vi "MIC.vi"() -> ()   [LabVIEW 2022 SP3]
uses:
  <vilib>/Analysis/3filter.llb/Filter Passband Type.ctl
  <vilib>/DAQmx/read.llb/DAQmx Read (Analog 1D Wfm NChan NSamp).vi
  <vilib>/DAQmx/write.llb/DAQmx Write (Analog 1D DBL NChan 1Samp).vi
  <vilib>/DAQmx/create/channels.llb/DAQmx Create Channel (AI-Voltage-Basic).vi
  <vilib>/DAQmx/configure/timing.llb/DAQmx Timing (Sample Clock).vi
  <vilib>/DAQmx/create/channels.llb/DAQmx Create Channel (AO-Voltage-Basic).vi
  <vilib>/DAQmx/miscellaneous.llb/DAQmx Fill In Error Info.vi
  <vilib>/Analysis/3filter.llb/Butterworth Filter (DBL).vi
  <vilib>/Analysis/NI_AALBase.lvlib
panel:
  out "Inverted Signal":dbl[](graph)
  out "Y":dbl[](array[numeric])
  in  "stop":bool
  out "Filtered":dbl[](graph)
  out "Filtered X":dbl[](array[numeric])
  out "INput":dbl[](graph)
  out "data":waveform(dbl)
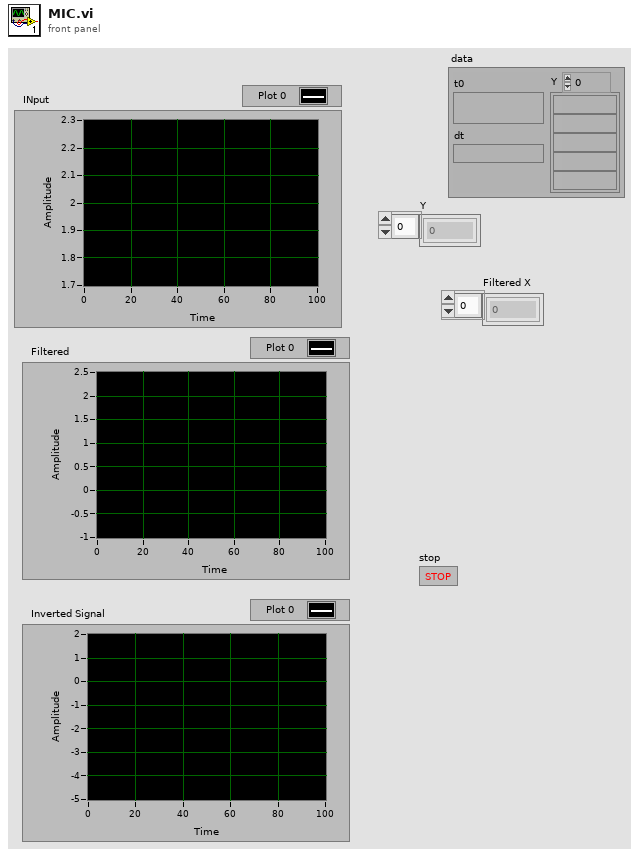
[diagram p1: front panel]
types:
  T1 = typedef "NI_AALBase.lvlib/Filter Passband Type.ctl" = enum32{"Lowpass", "Highpass", "Bandpass", "Bandstop"}
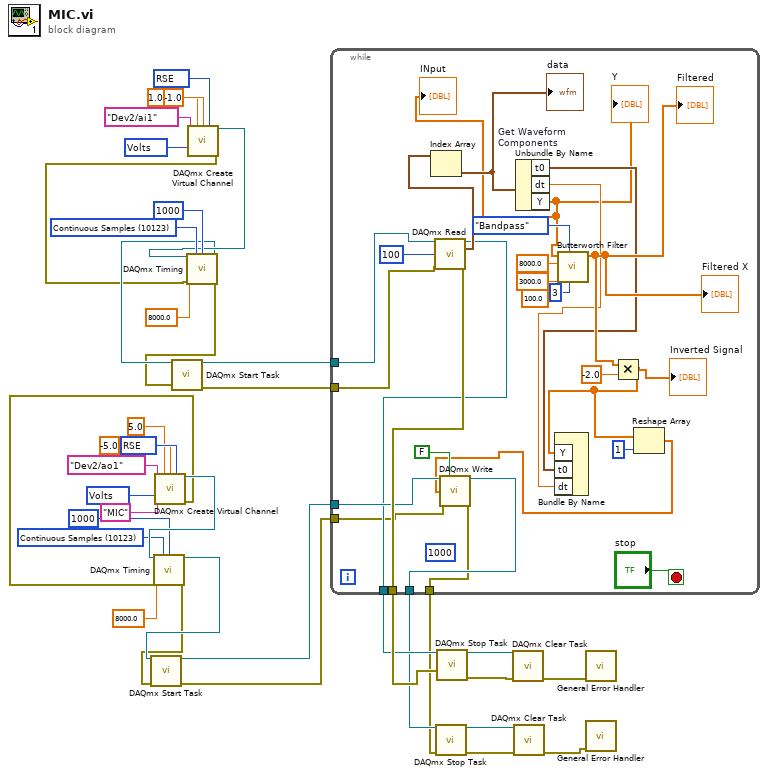
[diagram p0: block diagram]
diagram:
  w14 = 10123 items=["Finite Samples"=10178, "Continuous Samples"=10123, "Hardware Timed Single Point"=12522] ("sample mode")
  w18 = 10083 items=["Default"=-1, "RSE"=10083, "Differential"=10106, "Pseudodifferential"=12529] ("output terminal configuration")
  w20 = 10348 items=["Volts"=10348, "From Custom Scale"=10065] ("units")
  w32 = 10083 items=["Default"=-1, "RSE"=10083, "NRSE"=10078, "Differential"=10106, "Pseudodifferential"=12529] ("input terminal configuration")
  w33 = 10348 items=["Volts"=10348, "From Custom Scale"=10065] ("units")
  w35 = 10123 items=["Finite Samples"=10178, "Continuous Samples"=10123, "Hardware Timed Single Point"=12522] ("sample mode")
  n1 = call-poly <vilib>:"DAQmx Create Virtual Channel.vi"("maximum value"=5.0, "minimum value"=-5.0, "output terminal configuration"=w18, "physical channels"=tag "Dev2/ao1", "name to assign"="MIC", "units"=w20) -> ("task out"=w15:refnum<k21>, "error out"=w11:errorcluster)  [unwired: 8 in]
  n2 = call-poly <vilib>:"DAQmx Timing.vi"("task/channels in"=w15, "sample mode"=w14, "samples per channel"=1000, "rate"=8000.0, "error in"=w11) -> ("task out"=w10:refnum<k21>, "error out"=w5:errorcluster)  [unwired: 9 in]
  n3 = call <vilib>:"DAQmx Start Task.vi"("task/channels in"=w10, "error in"=w5) -> ("task out"=w9:refnum<k21>, "error out"=w4:errorcluster)  [unwired: 12 in]
  n4 = call-poly <vilib>:"DAQmx Create Virtual Channel.vi"("maximum value"=1.0, "minimum value"=-1.0, "input terminal configuration"=w32, "physical channels"=tag "Dev2/ai1", "units"=w33) -> ("task out"=w31:refnum<k21>, "error out"=w27:errorcluster)  [unwired: 9 in]
  n5 = call-poly <vilib>:"DAQmx Timing.vi"("task/channels in"=w31, "sample mode"=w35, "samples per channel"=1000, "rate"=8000.0, "error in"=w27) -> ("task out"=w29:refnum<k21>, "error out"=w26:errorcluster)  [unwired: 9 in]
  n6 = call <vilib>:"DAQmx Start Task.vi"("task/channels in"=w29, "error in"=w26) -> ("task out"=w28:refnum<k21>, "error out"=w25:errorcluster)  [unwired: 12 in]
  n7 = while {
    tunnel: w28 -> [w64]
    tunnel: w25 -> [w63]
    tunnel: [w62] -> w24
    tunnel: w9 -> [w53]
    tunnel: [w52] -> w8
    tunnel: [w51] -> w6
    tunnel: w4 -> [w50]
    tunnel: [w49] -> w3
    stop <- "stop" stop-if-true
    (unwired) u32 1000 ("number of samples written per channel")
    n8 = call-poly <vilib>:"DAQmx Read.vi"("task/channels in"=w64, "number of samples per channel"=100, "error in"=w63) -> ("task out"=w52:refnum<k21>, "data"=w61:waveform(dbl)[], "error out"=w62:errorcluster)  [unwired: 10 in]
    n9 = Index Array(array=w61) -> (element=w60:waveform(dbl))  [unwired: 1 in]
    "data" <- w60
    n10 = Unbundle By Name "Get Waveform Components"(w60) -> ("t0"=w46:timestamp, "dt"=w45:dbl, "Y"=w43:dbl[])
    "INput" <- w43
    "Y" <- w43
    n11 = call-poly <vilib>:"Butterworth Filter.vi"("order"=3, "filter type"=Filter_Passband_Type."Bandpass", "low cutoff freq: fl"=100.0, "high cutoff freq: fh"=3000.0, "sampling freq: fs"=8000.0, "X"=w43) -> ("Filtered X"=w47:dbl[])  [unwired: 2 in, 1 out]
    "Filtered X" <- w47
    "Filtered" <- w47
    n12 = Multiply(x=w47, y=-2.0) -> (x*y=w42:dbl[])
    "Inverted Signal" <- w42
    n13 = Bundle By Name("Y"=w42, "t0"=w46, "dt"=w45) -> ()  [unwired: 1 in, 1 out]
    n14 = Reshape Array(w42, 1 ("dimension size")) -> (w41:dbl[])
    n15 = call-poly <vilib>:"DAQmx Write.vi"("task/channels in"=w53, "auto start"=FALSE, "data"=w41, "error in"=w50) -> ("task out"=w51:refnum<k21>, "error out"=w49:errorcluster)  [unwired: 9 in, 1 out]
  }
  n16 = call <vilib>:"DAQmx Stop Task.vi"("task/channels in"=w6, "error in"=w3) -> ("task out"=w7:refnum<k21>, "error out"=w2:errorcluster)  [unwired: 12 in]
  n17 = call <vilib>:"DAQmx Stop Task.vi"("task/channels in"=w8, "error in"=w24) -> ("task out"=w30:refnum<k21>, "error out"=w23:errorcluster)  [unwired: 12 in]
  n18 = call <vilib>:"DAQmx Clear Task.vi"("task in"=w30, "error in"=w23) -> ("error out"=w22:errorcluster)  [unwired: 13 in]
  n19 = call <vilib>:"DAQmx Clear Task.vi"("task in"=w7, "error in"=w2) -> ("error out"=w1:errorcluster)  [unwired: 13 in]
  n20 = call <vilib>:"General Error Handler.vi"("error in (no error)"=w22) -> ()  [unwired: 10 in, 5 out]
  n21 = call <vilib>:"General Error Handler.vi"("error in (no error)"=w1) -> ()  [unwired: 10 in, 5 out]
